vi "Housekeeping.vi"(8 "error in (no error)":errorcluster, 10 "Force Refresh":bool, 11 "CIFChannelMng in":refnum<class "CIFChannelMng.lvclass">) -> (0 "error out":errorcluster, 3 "CIFChannelMng out":refnum<class "CIFChannelMng.lvclass">)   [LabVIEW 2021, in "CIFChannelMng.lvclass"]
uses:
  CIFChannelMng.lvclass
  CIFChannelMng.lvclass/CIFChannelMng.ctl
  <vilib>/CIF Foundation/CIF Out of Band Commands/CIFOutOfBand.lvclass/CIFOutOfBand.ctl
  OOB/OOB_Rx/ChanMngOOB_Rx.lvclass/ChanMngOOB_Rx.ctl
  <vilib>/CIF Foundation/CIF Channels Core/CIFChannels/CIFChannels.lvclass/CIFChannels.ctl
  <vilib>/CIF Foundation/CIF Out of Band Commands/Read Commands.vi
  OOB/OOB_Rx/Private/Command Settings.vi
  OOB/OOB_Rx/Private/Read Payload.vi
  Utilities/Get Channel Index by Name.vi
  <vilib>/CIF Foundation/CIF Channels Core/CIFChannels/Accessors/Read Tag Forced.vi
  <vilib>/CIF Foundation/CIF Channels Core/CIFChannels/Accessors/Read Channel State.vi
  SubVIs/Add Error Channel Manager.vi
  <vilib>/CIF Foundation/CIF Out of Band Commands/Queue Command.vi
  <vilib>/CIF Foundation/CIF Out of Band Commands/Utilities/Command to Bitwise Command.vi
  <vilib>/CIF Foundation/CIF Out of Band Commands/Accessors/Read Local OOB Data.vi
  SubVIs/Get Original FIFO Channel Name.vi
  <vilib>/CIF Foundation/CIF Channels Core/ChannelCommon/Utilities/Add Error.vi
  <vilib>/CIF Foundation/CIF Utilities/Errors/Append Error Location.vi
  OOB/OOB_Rx/ChanMngOOB_Rx.lvclass
  C:/Program Files/National Instruments/LabVIEW 2021/vi.lib/CIF Foundation/CIF Out of Band Commands/CIFOutOfBand.lvclass
  OOB/OOB_Tx/ChnMngOOB_Tx.lvclass
  <vilib>/CIF Foundation/CIF Channels Core/CIFChannels/Core/Set Force.vi
  <vilib>/CIF Foundation/CIF Channels Core/CIFChannels/CIFChannels.lvclass
  <vilib>/CIF Foundation/CIF Out of Band Commands/CIFOutOfBand.lvclass
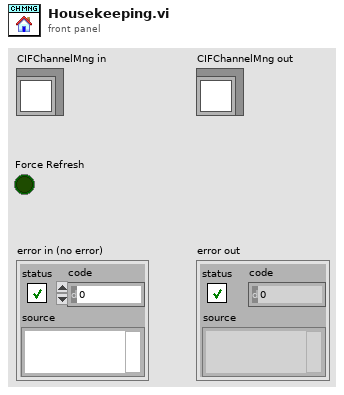
[diagram p1: front panel]
types:
  T1 = typedef "ChanMngOOB_Rx.lvclass/OOB ChnMng Commands.ctl" = enum8{"Connect Channel", "Force Channel", "Add FIFO Pub", "Remove FIFO Pub"}
  T2 = typedef "ChanMngOOB_Rx.lvclass/Channel Fault Data.ctl" = cluster{"Channel Name":string, "Force Data":u8[], "Force Active":bool}
  T3 = typedef "ChanMngOOB_Rx.lvclass/Channel Connection Data.ctl" = cluster{"Publisher Name":string, "Subscriber Name":string, "Connection Data":u8[]}
  T4 = typedef "ChanMngOOB_Rx.lvclass/FIFO Publisher.ctl" = cluster{"Publisher Name":string, "New FIFO Instance Config":T5}
  T5 = typedef "ChannelCommon.lvlib/New FIFO Instance Configuration.ctl" = cluster{"Primary":bool, "Backpressure":bool, "Message/FIFO Override":u32}
  T6 = typedef "ChnMngOOB_Tx.lvclass/FIFO Publisher Return.ctl" = cluster{"FIFO Pub Name":string, "error":errorcluster, "Added":bool}
  T7 = typedef "CIFChannelMng.lvclass/Channel List for OOB.ctl" = cluster{"Name":string, "Direction":T8, "Type":string, "Connected?":bool, "Connected Name":string, "Custom Config Data":u8[], "Forced?":bool, "Multi-Writer":bool}
  T8 = typedef "CIFChannels.lvclass/Direction.ctl" = enum16{"Publisher", "Subscriber"}
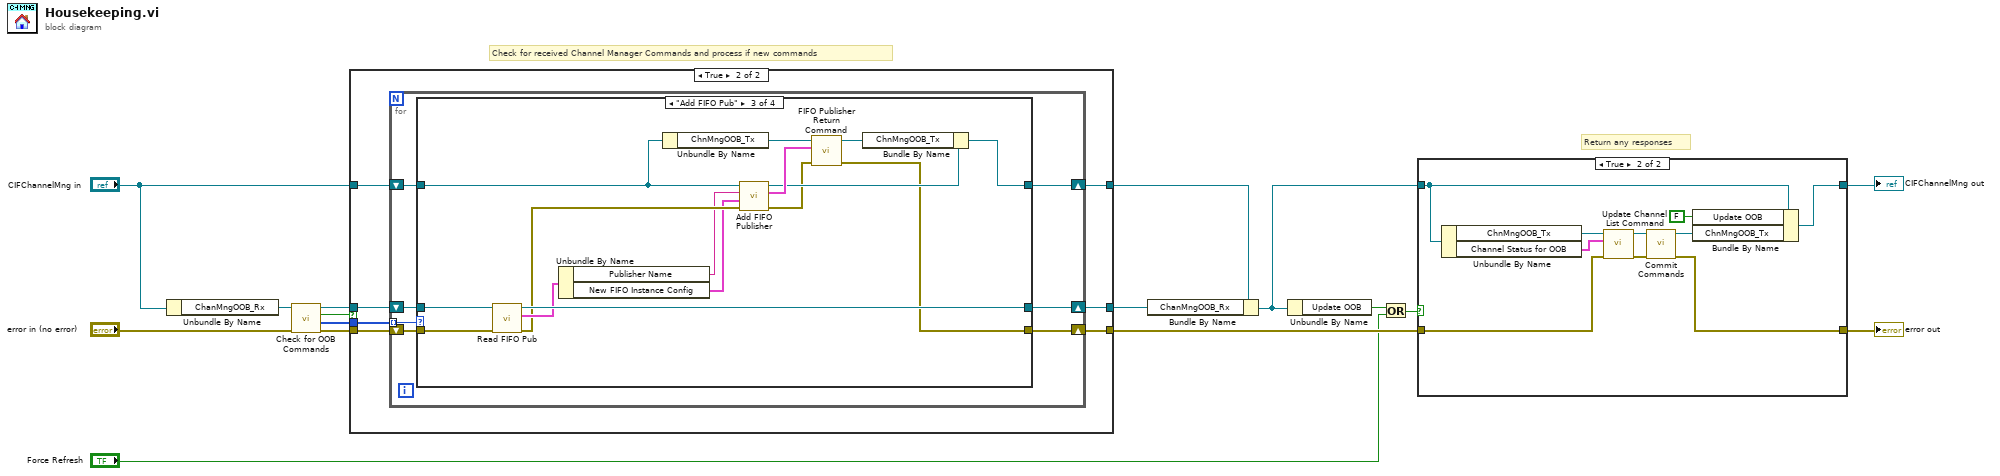
[diagram p0: block diagram]
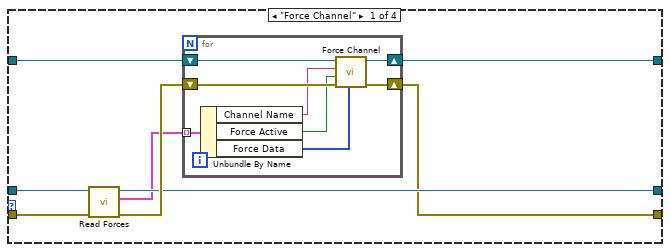
[diagram p4: hidden frame]
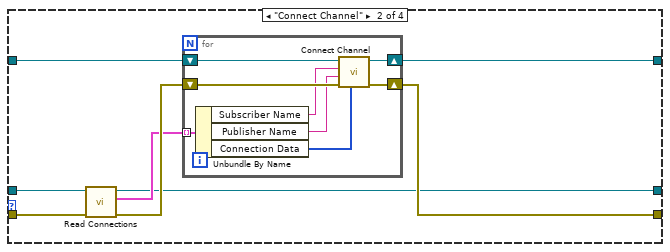
[diagram p5: hidden frame]
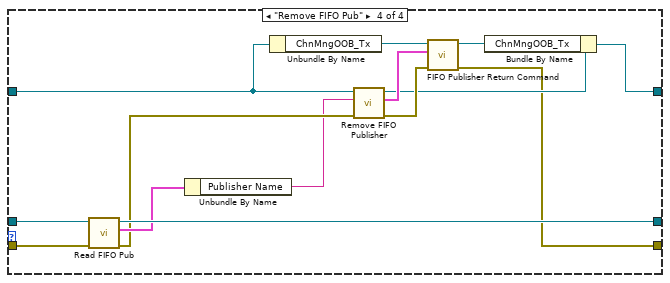
[diagram p6: hidden frame]
diagram:
  # "Return any responses"
  # "Check for received Channel Manager Commands and process if new commands"
  n1 = Unbundle By Name("CIFChannelMng in") -> ("ChanMngOOB_Rx"=w16:refnum<class "ChanMngOOB_Rx.lvclass">)
  n2 = call "Check for OOB Commands.vi"("error in (no error)"="error in (no error)", "ChanMngOOB_Rx in"=w16) -> ("error out"=w11:errorcluster, "Commands"=w13:T1[], "New Commands"=w14:bool, "ChanMngOOB_Rx out"=w12:refnum<class "ChanMngOOB_Rx.lvclass">)  [unwired: 6 in]
  n3 = case shown="True" w14 {
    tunnel: w13 -> [_ w26]
    tunnel: w12 -> [w18 w25]
    tunnel: w11 -> [w17 w24]
    tunnel: "CIFChannelMng in" -> [w19 w23]
    tunnel: [w17 w22] -> w6
    tunnel: [w19 w21] -> w10
    tunnel: [w18 w20] -> w9
    frame False {
    }
    frame True {
      n4 = for {
        tunnel: w26 -> [w33] mode=indexing
        shift-right: [w29] -> w20
        shift-left: w25 -> [w32]
        shift-right: [w28] -> w21
        shift-left: w23 -> [w30]
        shift-right: [w27] -> w22
        shift-left: w24 -> [w31]
        n5 = case shown="\"Add FIFO Pub\"" w33 {
          tunnel: w32 -> [w41 w54 w79 w93]
          tunnel: w31 -> [w40 w53 w80 w94]
          tunnel: w30 -> [w39 w57 w73 w88]
          tunnel: [w37 w50 w78 w92] -> w29
          tunnel: [w35 w56 w69 w89] -> w28
          tunnel: [w34 w55 w66 w81] -> w27
          frame "Force Channel" {
            n6 = call "Read Forces.vi"("error in"=w40, "ChanMngOOB_Rx in"=w41) -> ("error out"=w38:errorcluster, "Forces"=w36:T2[], "ChanMngOOB_Rx out"=w37:refnum<class "ChanMngOOB_Rx.lvclass">)  [unwired: 6 in, 1 out]
            n7 = for {
              tunnel: w36 -> [w47] mode=indexing
              shift-right: [w43] -> w35
              shift-left: w39 -> [w49]
              shift-right: [w42] -> w34
              shift-left: w38 -> [w48]
              n8 = Unbundle By Name(w47) -> ("Channel Name"=w46:string, "Force Active"=w45:bool, "Force Data"=w44:u8[])
              n9 = call "Force Channel.vi"("Force Data"=w44, "error in (no error)"=w48, "Force Active"=w45, "Channel Name"=w46, "CIFChannelMng in"=w49) -> ("error out"=w42:errorcluster, "CIFChannelMng out"=w43:refnum<class "CIFChannelMng.lvclass">)  [unwired: 5 in]
            }
          }
          frame "Connect Channel" {
            n10 = call "Read Connections.vi"("error in"=w53, "ChanMngOOB_Rx in"=w54) -> ("error out"=w52:errorcluster, "Connections"=w51:T3[], "ChanMngOOB_Rx out"=w50:refnum<class "ChanMngOOB_Rx.lvclass">)  [unwired: 6 in, 1 out]
            n11 = for {
              tunnel: w51 -> [w65] mode=indexing
              shift-right: [w63] -> w56
              shift-left: w57 -> [w64]
              shift-right: [w62] -> w55
              shift-left: w52 -> [w61]
              n12 = Unbundle By Name(w65) -> ("Subscriber Name"=w60:string, "Publisher Name"=w59:string, "Connection Data"=w58:u8[])
              n13 = call "Connect Channel.vi"("Custom Channel Config Data"=w58, "error in (no error)"=w61, "Publisher Name"=w59, "Subscriber Name"=w60, "CIFChannelMng in"=w64) -> ("error out"=w62:errorcluster, "CIFChannelMng out"=w63:refnum<class "CIFChannelMng.lvclass">)  [unwired: 5 in]
            }
          }
          frame "Add FIFO Pub" {
            n14 = call "Read FIFO Pub.vi"("error in"=w80, "ChanMngOOB_Rx in"=w79) -> ("error out"=w76:errorcluster, "FIFO Pub"=w77:T4, "ChanMngOOB_Rx out"=w78:refnum<class "ChanMngOOB_Rx.lvclass">)  [unwired: 7 in]
            n15 = Unbundle By Name(w77) -> ("Publisher Name"=w74:string, "New FIFO Instance Config"=w75:T5)
            n16 = Unbundle By Name(w73) -> ("ChnMngOOB_Tx"=w72:refnum<class "ChnMngOOB_Tx.lvclass">)
            n17 = call "Add FIFO Publisher.vi"("error in (no error)"=w76, "New FIFO Instance Config"=w75, "Channel Name"=w74, "CIFChannelMng in"=w73) -> ("error out"=w68:errorcluster, "FIFO Publisher"=w71:T6, "CIFChannelMng out"=w70:refnum<class "CIFChannelMng.lvclass">)  [unwired: 5 in]
            n18 = call "FIFO Publisher Return Command.vi"("error in"=w68, "FIFO Publisher"=w71, "ChanMngOOB_Tx in"=w72) -> ("error out"=w66:errorcluster, "ChanMngOOB_Tx out"=w67:refnum<class "ChnMngOOB_Tx.lvclass">)  [unwired: 7 in]
            n19 = Bundle By Name(cluster=w70, "ChnMngOOB_Tx"=w67) -> (w69:refnum<class "CIFChannelMng.lvclass">)
          }
          frame "Remove FIFO Pub" {
            n20 = call "Read FIFO Pub.vi"("error in"=w94, "ChanMngOOB_Rx in"=w93) -> ("error out"=w87:errorcluster, "FIFO Pub"=w91:T4, "ChanMngOOB_Rx out"=w92:refnum<class "ChanMngOOB_Rx.lvclass">)  [unwired: 7 in]
            n21 = Unbundle By Name(w91) -> ("Publisher Name"=w86:string)
            n22 = Unbundle By Name(w88) -> ("ChnMngOOB_Tx"=w90:refnum<class "ChnMngOOB_Tx.lvclass">)
            n23 = call "Remove FIFO Publisher.vi"("error in (no error)"=w87, "Channel Name"=w86, "CIFChannelMng in"=w88) -> ("error out"=w85:errorcluster, "FIFO Publisher"=w84:T6, "CIFChannelMng out"=w83:refnum<class "CIFChannelMng.lvclass">)  [unwired: 6 in]
            n24 = call "FIFO Publisher Return Command.vi"("error in"=w85, "FIFO Publisher"=w84, "ChanMngOOB_Tx in"=w90) -> ("error out"=w81:errorcluster, "ChanMngOOB_Tx out"=w82:refnum<class "ChnMngOOB_Tx.lvclass">)  [unwired: 7 in]
            n25 = Bundle By Name(cluster=w83, "ChnMngOOB_Tx"=w82) -> (w89:refnum<class "CIFChannelMng.lvclass">)
          }
        }
      }
    }
  }
  n26 = Bundle By Name(cluster=w10, "ChanMngOOB_Rx"=w9) -> (w7:refnum<class "CIFChannelMng.lvclass">)
  n27 = Unbundle By Name(w7) -> ("Update OOB"=w3:bool)
  n28 = Or(x=w3, y="Force Refresh") -> (x .or. y?=w2:bool)
  n29 = case shown="True" w2 {
    tunnel: w7 -> [w95 w99]
    tunnel: w6 -> [w96 w104]
    tunnel: [w95 w98] -> w5
    tunnel: [w96 w97] -> w4
    frame False {
    }
    frame True {
      n30 = Unbundle By Name(w99) -> ("ChnMngOOB_Tx"=w106:refnum<class "ChnMngOOB_Tx.lvclass">, "Channel Status for OOB"=w105:T7[])
      n31 = call "Update Channel List Command.vi"("error in"=w104, "Channel List"=w105, "ChanMngOOB_Tx in"=w106) -> ("error out"=w102:errorcluster, "ChanMngOOB_Tx out"=w103:refnum<class "ChnMngOOB_Tx.lvclass">)  [unwired: 7 in]
      n32 = call <vilib>:"Commit Commands.vi"("error in"=w102, "OOB in"=w103) -> ("error out"=w97:errorcluster, "OOB out"=w101:refnum<class "ChnMngOOB_Tx.lvclass">)  [unwired: 8 in]
      n33 = Bundle By Name(cluster=w99, "Update OOB"=FALSE, "ChnMngOOB_Tx"=w101) -> (w98:refnum<class "CIFChannelMng.lvclass">)
    }
  }
  "error out" <- w4
  "CIFChannelMng out" <- w5
